vi "HEWH Timer Resetter.vi"(8 "Error In":errorcluster, 10 "Set Status":bool=TRUE, 11 "Station ID in":T1) -> (0 "Error Out":errorcluster)   [LabVIEW 2019]
uses:
  Custom Instrument Control/MW100/Type Definitions/Station ID Selector.ctl
  Utility/Type Definitions/UTILITY Notifier.ctl
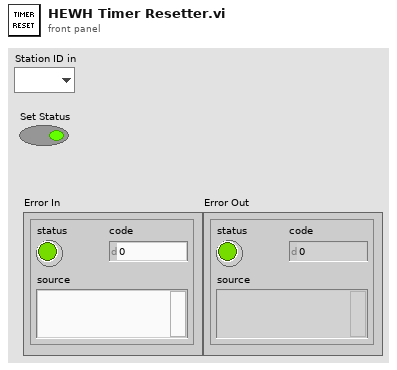
[diagram p1: front panel]
types:
  T1 = typedef "Station ID Selector.ctl" = enum16{"", "A", "B", "C", "D", "Global"}
  T2 = typedef "UTILITY Notifier.ctl" = enum16{"Set", "Read", "Release Ref"}
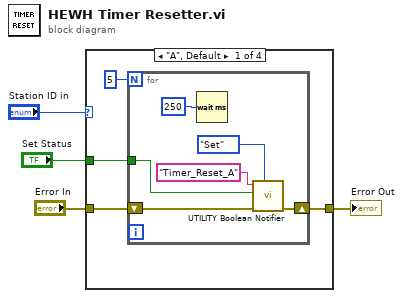
[diagram p0: block diagram]
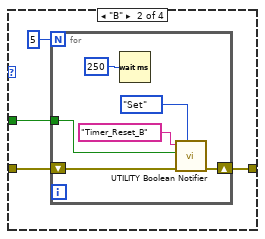
[diagram p2: hidden frame]
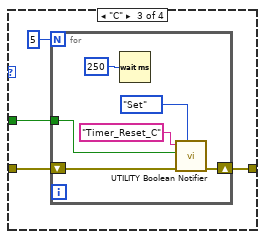
[diagram p3: hidden frame]
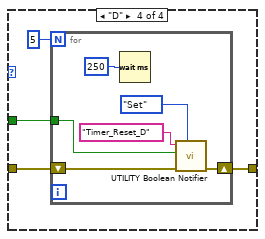
[diagram p4: hidden frame]
diagram:
  n1 = case shown="\"A\", Default" "Station ID in" {
    tunnel: "Set Status" -> [w7 w17 w27 w37]
    tunnel: "Error In" -> [w6 w16 w26 w36]
    tunnel: [w5 w15 w25 w35] -> w1
    frame "A", Default {
      n2 = for {
        N: 5 -> [_]
        shift-right: [w9] -> w5
        shift-left: w6 -> [w10]
        tunnel: w7 -> [w11]
        n3 = Wait (ms)(milliseconds to wait=u32 250) -> ()  [unwired: 1 out]
        n4 = call "UTILITY Boolean Notifier.vi"("Status"=UTILITY_Notifier."Set", "error in (no error)"=w10, "Set Status"=w11, "name (unnamed)"="Timer_Reset_A") -> ("error out"=w9:errorcluster)  [unwired: 6 in, 1 out]
      }
    }
    frame "B" {
      n5 = for {
        N: 5 -> [_]
        shift-right: [w19] -> w15
        shift-left: w16 -> [w20]
        tunnel: w17 -> [w21]
        n6 = Wait (ms)(milliseconds to wait=u32 250) -> ()  [unwired: 1 out]
        n7 = call "UTILITY Boolean Notifier.vi"("Status"=UTILITY_Notifier."Set", "error in (no error)"=w20, "Set Status"=w21, "name (unnamed)"="Timer_Reset_B") -> ("error out"=w19:errorcluster)  [unwired: 6 in, 1 out]
      }
    }
    frame "C" {
      n8 = for {
        N: 5 -> [_]
        shift-right: [w29] -> w25
        shift-left: w26 -> [w30]
        tunnel: w27 -> [w31]
        n9 = Wait (ms)(milliseconds to wait=u32 250) -> ()  [unwired: 1 out]
        n10 = call "UTILITY Boolean Notifier.vi"("Status"=UTILITY_Notifier."Set", "error in (no error)"=w30, "Set Status"=w31, "name (unnamed)"="Timer_Reset_C") -> ("error out"=w29:errorcluster)  [unwired: 6 in, 1 out]
      }
    }
    frame "D" {
      n11 = for {
        N: 5 -> [_]
        shift-right: [w39] -> w35
        shift-left: w36 -> [w40]
        tunnel: w37 -> [w41]
        n12 = Wait (ms)(milliseconds to wait=u32 250) -> ()  [unwired: 1 out]
        n13 = call "UTILITY Boolean Notifier.vi"("Status"=UTILITY_Notifier."Set", "error in (no error)"=w40, "Set Status"=w41, "name (unnamed)"="Timer_Reset_D") -> ("error out"=w39:errorcluster)  [unwired: 6 in, 1 out]
      }
    }
  }
  "Error Out" <- w1
